vi "svx_SC Line IndexToCheckbox.vi"(4 "All Children Tags":string[](array[string]), 10 "RowIdx":i32, 11 "Tree ref in":refnum<vi>) -> (3 "Tree ref out":refnum<vi>)   [LabVIEW 2017, in "SVX SC Line.xctl"]
uses:
  <vilib>/addons/_XControls/Shaft Centerline/SVX SC Line.xctl
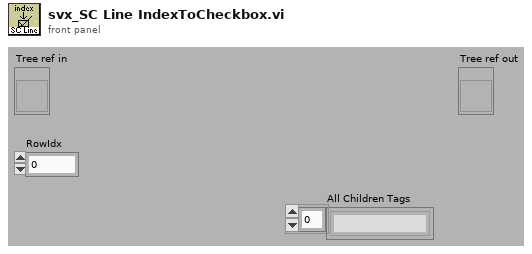
[diagram p1: front panel]
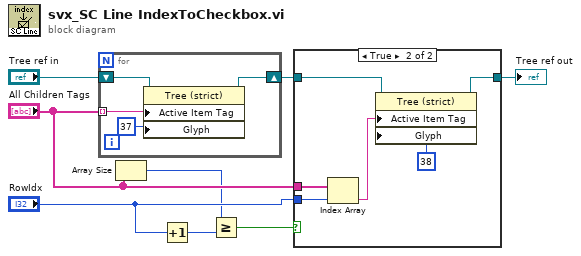
[diagram p0: block diagram]
diagram:
  n1 = for {
    tunnel: "All Children Tags" -> [w11] mode=indexing
    shift-right: [w9] -> w7
    shift-left: "Tree ref in" -> [w12]
    n2 = property class="Tree (strict)"(reference=w12, "Active Item Tag"=w11, "Glyph"=37 ("Active Item:Symbol Index")) -> (reference out=w9:refnum<vi>)  [unwired: 1 in, 1 out]
  }
  n3 = Array Size(array="All Children Tags") -> (size(s)=w3:i32)
  n4 = Increment(x="RowIdx") -> (x+1=w2:i32)
  n5 = Greater Or Equal?(x=w3, y=w2) -> (x >= y?=w1:bool)
  n6 = case shown="True" w1 {
    tunnel: w7 -> [w13 w19]
    tunnel: [w13 w16] -> w6
    tunnel: "All Children Tags" -> [_ w15]
    tunnel: "RowIdx" -> [_ w14]
    frame False {
    }
    frame True {
      n7 = Index Array(array=w15, index=w14) -> (element=w18:string)
      n8 = property class="Tree (strict)"(reference=w19, "Active Item Tag"=w18, "Glyph"=38 ("Active Item:Symbol Index")) -> (reference out=w16:refnum<vi>)  [unwired: 1 in, 1 out]
    }
  }
  "Tree ref out" <- w6
